vi "9219_MatchChannelConfig.vi"(1 "ConfigTD in":T1 {"Conversion Time" items=["High Speed", "Best 60 Hz Rejection", "Best 50 Hz Rejection", "High Resolution"]; "TCoupleType" items=["J", "K", "T", "E", "R", "S", "N", "B"]; "DegreeRange" items=["Raw units", "Degrees Kelvin", "Degrees Celsius", "Degrees Fahrenheit", "Degrees Rankine"]; "RtdType" items=["TCR3851"=1, "TCR3750"=2, "TCR3916"=3, "TCR3920"=4, "TCR3911"=5, "TCR3928"=6, "Custom"=0]}, 4 "Selected Channels":i32[](array[numeric])) -> (7 "Type RTD":u8, 8 "Valid mode?":bool, 9 "Valid RTD?":bool, 10 "CVD":dbl[](array[numeric]), 11 "Vald CVD":bool[](array[boolean]), 12 "Mode value":u8, 13 "Valid range2?":bool, 14 "Valid range?":bool, 15 "Range value":u8, 16 "Valid threshold?":bool, 18 "Threshold value":dbl min=0.0 max=60.0 step=9.99999993922529e-09 format="%#.8f", 19 "Type range2":u8)   [LabVIEW 2020, in "Modules.lvlib" / "9219.lvclass"]
uses:
  9219.lvclass
  9219 Config.ctl
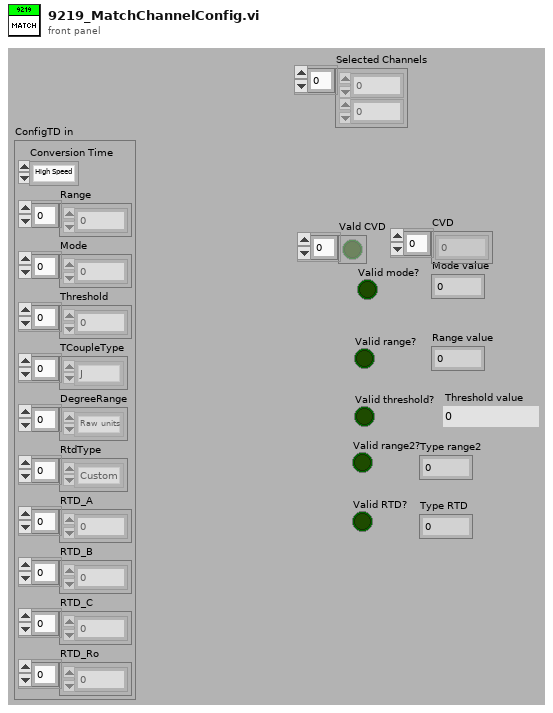
[diagram p1: front panel]
types:
  T1 = typedef "Modules.lvlib/9219.lvclass/9219 Config.ctl" = cluster{"Conversion Time":u16, "Range":u8[], "Mode":u8[], "Threshold":dbl[], "TCoupleType":u8[], "DegreeRange":u8[], "RtdType":u8[], "RTD_A":dbl[], "RTD_B":dbl[], "RTD_C":dbl[], "RTD_Ro":dbl[]}
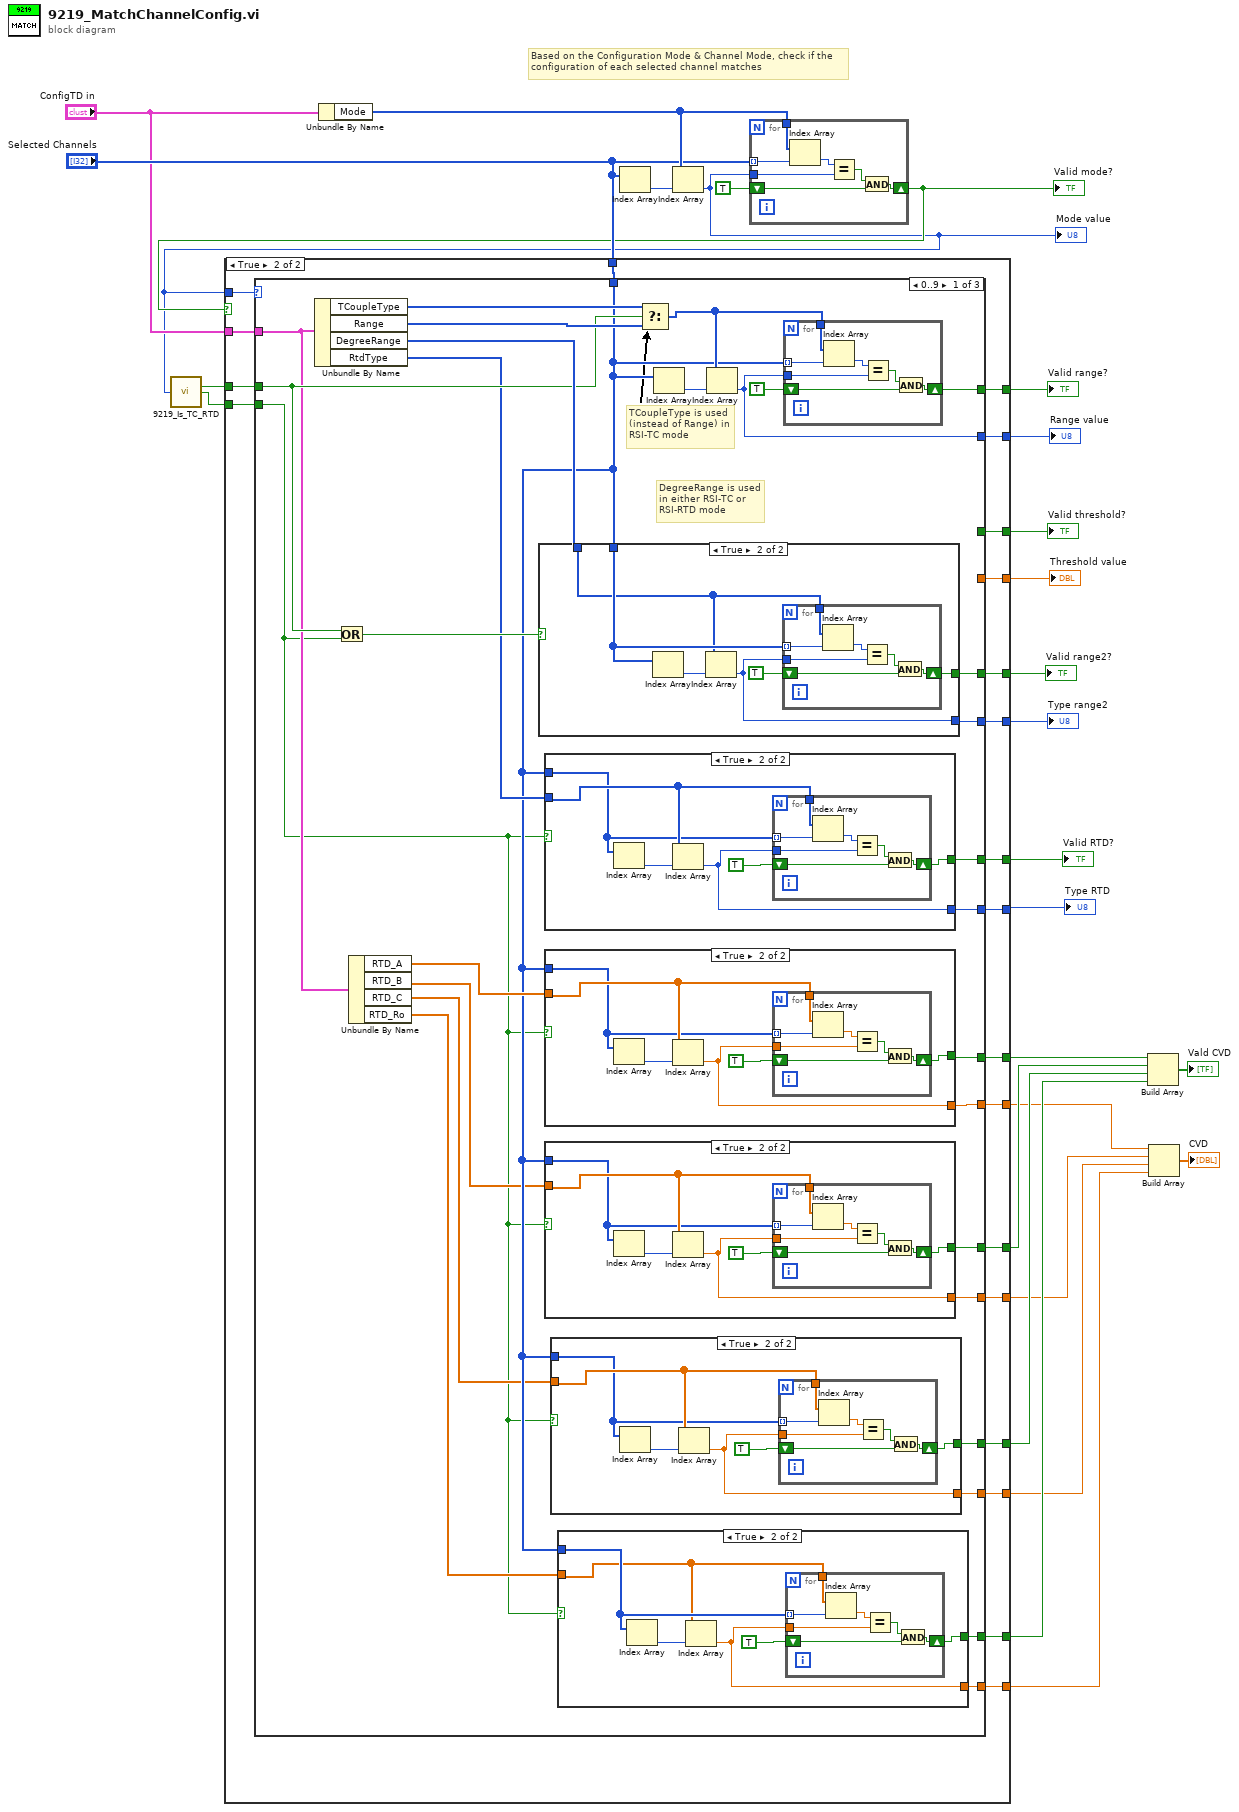
[diagram p0: block diagram]
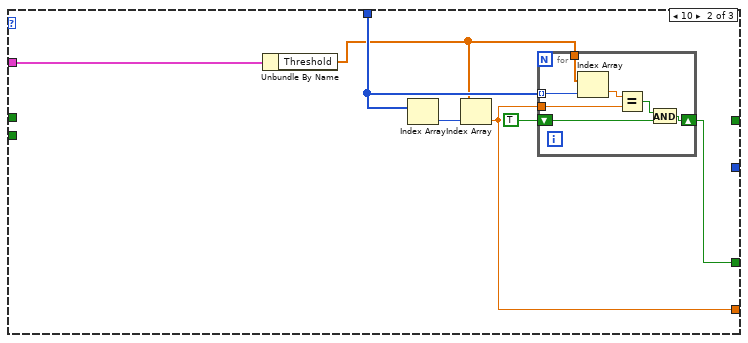
[diagram p9: hidden frame]
diagram:
  # "Based on the Configuration Mode & Channel Mode, check if the configuration of each selected channel matches"
  n1 = Unbundle By Name("ConfigTD in") -> ("Mode"=w23:u8[])
  n2 = Index Array(array="Selected Channels") -> (element=w25:i32)  [unwired: 1 in]
  n3 = Index Array(array=w23, index=w25) -> (element=w14:u8)
  "Mode value" <- w14
  n4 = call "9219_Is_TC_RTD.vi"("Mode"=w14) -> ("Is RIOScan / Thermocouple"=w15:bool, "Is RIOScan / RTD"=w13:bool)  [unwired: 13 in]
  n5 = for {
    tunnel: "Selected Channels" -> [w33] mode=indexing
    tunnel: w23 -> [w34]
    tunnel: w14 -> [w31]
    shift-right: [w29] -> w18
    shift-left: TRUE -> [w28]
    n6 = Index Array(array=w34, index=w33) -> (element=w32:u8)
    n7 = Equal?(x=w32, y=w31) -> (x = y?=w30:bool)
    n8 = And(x=w30, y=w28) -> (x .and. y?=w29:bool)
  }
  "Valid mode?" <- w18
  n9 = case shown="True" w18 {
    tunnel: [_ w55] -> w27
    tunnel: [_ w54] -> w26
    tunnel: "Selected Channels" -> [_ w53]
    tunnel: [_ w50] -> w21
    tunnel: [_ w49] -> w16
    tunnel: [_ w47] -> w20
    tunnel: [_ w48] -> w19
    tunnel: "ConfigTD in" -> [_ w52]
    tunnel: w14 -> [_ w51]
    tunnel: w15 -> [_ w46]
    tunnel: w13 -> [_ w45]
    tunnel: [_ w44] -> w11
    tunnel: [_ w43] -> w12
    tunnel: [_ w42] -> w10
    tunnel: [_ w41] -> w9
    tunnel: [_ w40] -> w8
    tunnel: [_ w39] -> w7
    tunnel: [_ w38] -> w6
    tunnel: [_ w37] -> w5
    tunnel: [_ w36] -> w4
    tunnel: [_ w35] -> w3
    frame False {
      # "Invalid mode - thus no other configurations are valid."
    }
    frame True {
      n10 = case shown="0..9" w51 {
        tunnel: [w82 _ _] -> w55
        tunnel: [w83 _ _] -> w54
        tunnel: w53 -> [w68 w175 _]
        tunnel: w52 -> [w70 w174 _]
        tunnel: [_ w172 _] -> w50
        tunnel: [_ w171 _] -> w49
        tunnel: [w80 _ _] -> w48
        tunnel: [w81 _ _] -> w47
        tunnel: w46 -> [w74 _ _]
        tunnel: w45 -> [w64 _ _]
        tunnel: [w72 _ _] -> w44
        tunnel: [w71 _ _] -> w43
        tunnel: [w63 _ _] -> w42
        tunnel: [w62 _ _] -> w41
        tunnel: [w61 _ _] -> w40
        tunnel: [w60 _ _] -> w39
        tunnel: [w59 _ _] -> w38
        tunnel: [w58 _ _] -> w37
        tunnel: [w57 _ _] -> w36
        tunnel: [w56 _ _] -> w35
        frame 0..9 {
          # "TCoupleType is used (instead of Range) in RSI-TC mode"
          # "DegreeRange is used in either RSI-TC or RSI-RTD mode"
          n11 = Unbundle By Name(w70) -> ("TCoupleType"=w77:u8[], "Range"=w76:u8[], "DegreeRange"=w79:u8[], "RtdType"=w73:u8[])
          n12 = Or(x=w74, y=w64) -> (x .or. y?=w75:bool)
          n13 = Unbundle By Name(w70) -> ("RTD_A"=w69:dbl[], "RTD_B"=w67:dbl[], "RTD_C"=w66:dbl[], "RTD_Ro"=w65:dbl[])
          n14 = case shown="True" w75 {
            tunnel: [_ w154] -> w81
            tunnel: [_ w153] -> w80
            tunnel: w68 -> [_ w152]
            tunnel: w79 -> [_ w151]
            frame False {
            }
            frame True {
              n15 = Index Array(array=w152) -> (element=w156:i32)  [unwired: 1 in]
              n16 = Index Array(array=w151, index=w156) -> (element=w154:u8)
              n17 = for {
                tunnel: w152 -> [w162] mode=indexing
                tunnel: w151 -> [w163]
                tunnel: w154 -> [w160]
                shift-right: [w158] -> w153
                shift-left: TRUE -> [w157]
                n18 = Index Array(array=w163, index=w162) -> (element=w161:u8)
                n19 = Equal?(x=w161, y=w160) -> (x = y?=w159:bool)
                n20 = And(x=w159, y=w157) -> (x .and. y?=w158:bool)
              }
            }
          }
          n21 = case shown="True" w64 {
            tunnel: w73 -> [_ w143]
            tunnel: w68 -> [_ w142]
            tunnel: [_ w139] -> w72
            tunnel: [_ w138] -> w71
            frame False {
            }
            frame True {
              n22 = Index Array(array=w142) -> (element=w141:i32)  [unwired: 1 in]
              n23 = Index Array(array=w143, index=w141) -> (element=w139:u8)
              n24 = for {
                tunnel: w142 -> [w149] mode=indexing
                tunnel: w143 -> [w150]
                tunnel: w139 -> [w147]
                shift-right: [w145] -> w138
                shift-left: TRUE -> [w144]
                n25 = Index Array(array=w150, index=w149) -> (element=w148:u8)
                n26 = Equal?(x=w148, y=w147) -> (x = y?=w146:bool)
                n27 = And(x=w146, y=w144) -> (x .and. y?=w145:bool)
              }
            }
          }
          n28 = case shown="True" w64 {
            tunnel: w69 -> [_ w130]
            tunnel: w68 -> [_ w129]
            tunnel: [_ w126] -> w59
            tunnel: [_ w125] -> w63
            frame False {
            }
            frame True {
              n29 = Index Array(array=w129) -> (element=w128:i32)  [unwired: 1 in]
              n30 = Index Array(array=w130, index=w128) -> (element=w126:dbl)
              n31 = for {
                tunnel: w129 -> [w136] mode=indexing
                tunnel: w130 -> [w137]
                tunnel: w126 -> [w134]
                shift-right: [w132] -> w125
                shift-left: TRUE -> [w131]
                n32 = Index Array(array=w137, index=w136) -> (element=w135:dbl)
                n33 = Equal?(x=w135, y=w134) -> (x = y?=w133:bool)
                n34 = And(x=w133, y=w131) -> (x .and. y?=w132:bool)
              }
            }
          }
          n35 = case shown="True" w64 {
            tunnel: w67 -> [_ w117]
            tunnel: w68 -> [_ w116]
            tunnel: [_ w113] -> w58
            tunnel: [_ w112] -> w62
            frame False {
            }
            frame True {
              n36 = Index Array(array=w116) -> (element=w115:i32)  [unwired: 1 in]
              n37 = Index Array(array=w117, index=w115) -> (element=w113:dbl)
              n38 = for {
                tunnel: w116 -> [w123] mode=indexing
                tunnel: w117 -> [w124]
                tunnel: w113 -> [w121]
                shift-right: [w119] -> w112
                shift-left: TRUE -> [w118]
                n39 = Index Array(array=w124, index=w123) -> (element=w122:dbl)
                n40 = Equal?(x=w122, y=w121) -> (x = y?=w120:bool)
                n41 = And(x=w120, y=w118) -> (x .and. y?=w119:bool)
              }
            }
          }
          n42 = case shown="True" w64 {
            tunnel: w66 -> [_ w104]
            tunnel: w68 -> [_ w103]
            tunnel: [_ w100] -> w57
            tunnel: [_ w99] -> w61
            frame False {
            }
            frame True {
              n43 = Index Array(array=w103) -> (element=w102:i32)  [unwired: 1 in]
              n44 = Index Array(array=w104, index=w102) -> (element=w100:dbl)
              n45 = for {
                tunnel: w103 -> [w110] mode=indexing
                tunnel: w104 -> [w111]
                tunnel: w100 -> [w108]
                shift-right: [w106] -> w99
                shift-left: TRUE -> [w105]
                n46 = Index Array(array=w111, index=w110) -> (element=w109:dbl)
                n47 = Equal?(x=w109, y=w108) -> (x = y?=w107:bool)
                n48 = And(x=w107, y=w105) -> (x .and. y?=w106:bool)
              }
            }
          }
          n49 = case shown="True" w64 {
            tunnel: w68 -> [_ w91]
            tunnel: [_ w88] -> w56
            tunnel: [_ w87] -> w60
            tunnel: w65 -> [_ w86]
            frame False {
            }
            frame True {
              n50 = Index Array(array=w91) -> (element=w90:i32)  [unwired: 1 in]
              n51 = Index Array(array=w86, index=w90) -> (element=w88:dbl)
              n52 = for {
                tunnel: w91 -> [w97] mode=indexing
                tunnel: w86 -> [w98]
                tunnel: w88 -> [w95]
                shift-right: [w93] -> w87
                shift-left: TRUE -> [w92]
                n53 = Index Array(array=w98, index=w97) -> (element=w96:dbl)
                n54 = Equal?(x=w96, y=w95) -> (x = y?=w94:bool)
                n55 = And(x=w94, y=w92) -> (x .and. y?=w93:bool)
              }
            }
          }
          n56 = Select(t=w77, s=w74, f=w76) -> (s? t:f=w78:u8[])
          n57 = Index Array(array=w68) -> (element=w84:i32)  [unwired: 1 in]
          n58 = Index Array(array=w78, index=w84) -> (element=w82:u8)
          n59 = for {
            tunnel: w68 -> [w169] mode=indexing
            tunnel: w78 -> [w170]
            tunnel: w82 -> [w167]
            shift-right: [w165] -> w83
            shift-left: TRUE -> [w164]
            n60 = Index Array(array=w170, index=w169) -> (element=w168:u8)
            n61 = Equal?(x=w168, y=w167) -> (x = y?=w166:bool)
            n62 = And(x=w166, y=w164) -> (x .and. y?=w165:bool)
          }
        }
        frame 10 {
          n63 = Unbundle By Name(w174) -> ("Threshold"=w173:dbl[])
          n64 = Index Array(array=w175) -> (element=w176:i32)  [unwired: 1 in]
          n65 = Index Array(array=w173, index=w176) -> (element=w171:dbl)
          n66 = for {
            tunnel: w175 -> [w183] mode=indexing
            tunnel: w173 -> [w184]
            tunnel: w171 -> [w181]
            shift-right: [w179] -> w172
            shift-left: TRUE -> [w178]
            n67 = Index Array(array=w184, index=w183) -> (element=w182:dbl)
            n68 = Equal?(x=w182, y=w181) -> (x = y?=w180:bool)
            n69 = And(x=w180, y=w178) -> (x .and. y?=w179:bool)
          }
        }
        frame 11, Default {
        }
      }
    }
  }
  "Range value" <- w27
  "Valid range?" <- w26
  "Valid threshold?" <- w21
  "Type range2" <- w20
  "Valid range2?" <- w19
  "Threshold value" <- w16
  "Type RTD" <- w11
  "Valid RTD?" <- w12
  n70 = Build Array(w10, w9, w8, w7) -> (→"Vald CVD":bool[])
  n71 = Build Array(w6, w5, w4, w3) -> (→"CVD":dbl[])
